vi "FY6900.vi"(4 "Error In":errorcluster, 7 "Command":T13) -> (0 "Error Out":errorcluster, 3 "Response":T11)   [LabVIEW 2018]
uses:
  MOKO_LabViewLibrary/MokoLowLevel/MokoLowLovelControl/MLLC_Command.ctl
  MOKO_LabViewLibrary/MokoLowLevel/MokoLowLovelControl/MLLC_Mode.ctl
  MOKO_LabViewLibrary/MokoLowLevel/MokoLowLovelControl/MLLC_Response.ctl
  MOKO_LabViewLibrary/MokoLowLevel/MokoLowLovelControl/MLLC_ConnectCluster.ctl
  MOKO_LabViewLibrary/MokoLowLevel/MokoLowLovelControl/MLLC_InterfaceType.ctl
  MOKO_LabViewLibrary/MokoLowLevel/MokoLowLovelControl/MLLC_OpenedSession.ctl
  MOKO_LabViewLibrary/MokoLowLevel/MokoLowLovelControl/MLLC_InterfaceSettings.ctl
  MOKO_LabViewLibrary/MokoLowLevel/MokoLowLovelControl/MLLC_InterfaceKind.ctl
  MOKO_LabViewLibrary/MokoLowLevel/MokoLowLovelControl/MLLC_DriverName.ctl
  MOKO_LabViewLibrary/MokoLowLevel/MokoLowLovelControl/MLLC_ResponseInit.ctl
  MOKO_LabViewLibrary/MokoLowLevel/MokoLowLovelControl/MLLC_Request.ctl
  MOKO_LabViewLibrary/MokoLowLevel/MokoLowLovelControl/MLLC_ErrorCode.ctl
  MOKO_LabViewLibrary/MokoLowLevel/MokoLowLovelControl/MLLC_Rs232Settings.ctl
panel:
  in  "Error Code":T1=5420
  in  "Request":T2="UMO"
  in  "ResponseInit":T3="FY6900"
  in  "Driver Name":T4="FY6900"
  in  "Settings":T10={"Saved Data"=variant, "Permanent data"={"Connect"={"InterfaceType"=enum."VISA", "OpenedSession"="", "InterfaceSettings"={"Interface"=enum."RS232", "EOS 4 read"=enum."LF (\\n)", "EOS 4 write"=enum."LF (\\n)", "TMO, ms"=2000, "Sett"=variant(cluster{"Baud Rate":u32, "Data Bits":u16, "Parity":u16, "Stop Bits":u16, "Flow Control":u16, "Eho":bool} {"Baud Rate"=75, "Data Bits"=0, "Parity"=0, "Stop Bits"=0, "Flow Control"=0, "Eho"=FALSE})}}}}
  in  "Mode":T12=enum."Check"
  # "FY6900"
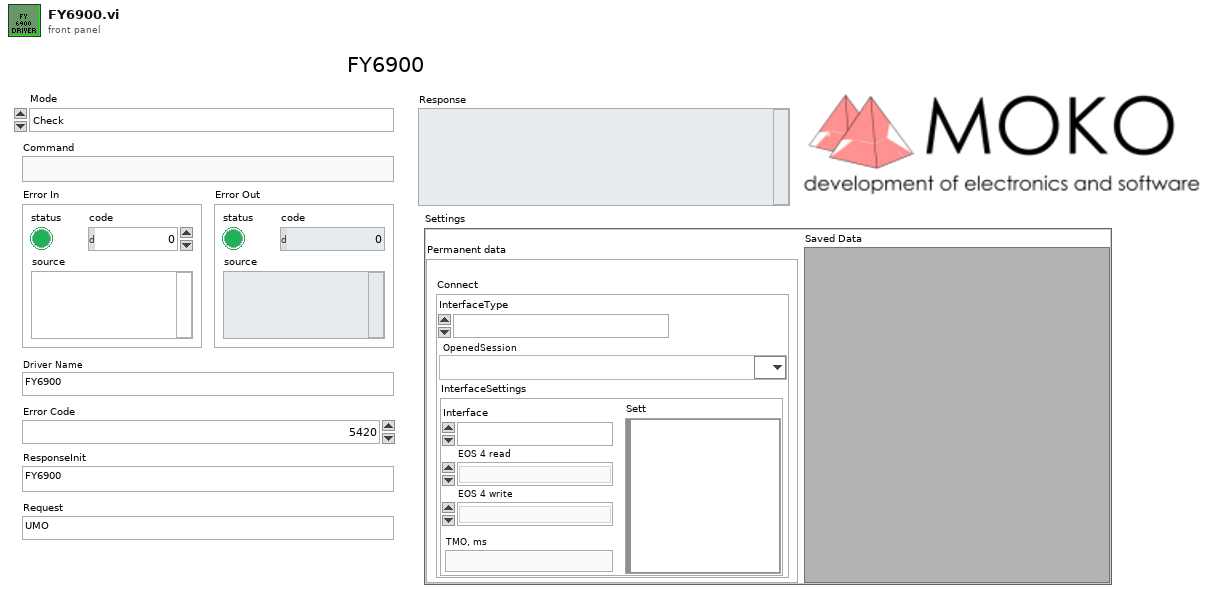
[diagram p1: front panel]
types:
  T1 = typedef "MLLC_ErrorCode.ctl" = u32
  T2 = typedef "MLLC_Request.ctl" = string
  T3 = typedef "MLLC_ResponseInit.ctl" = string
  T4 = typedef "MLLC_DriverName.ctl" = string
  T5 = typedef "MLLC_ConnectCluster.ctl" = cluster{"InterfaceType":T6, "OpenedSession":T7, "InterfaceSettings":T8}
  T6 = typedef "MLLC_InterfaceType.ctl" = enum16{"VISA", "Prologix USB-GPIB"}
  T7 = typedef "MLLC_OpenedSession.ctl" = refnum<visa-resource-name>
  T8 = typedef "MLLC_InterfaceSettings.ctl" = cluster{"Interface":T9, "EOS 4 read":enum16{"Default (=EOS 4 write)", "CR (\\r)", "LF (\\n)", "None"}, "EOS 4 write":enum16{"CR+LF (\\r\\n)", "CR (\\r)", "LF (\\n)", "None"}, "TMO, ms":i32, "Sett":variant}
  T9 = typedef "MLLC_InterfaceKind.ctl" = enum16{"RS232", "GPIB", "USB", "Ethernet", "another"}
  T10 = cluster{"Saved Data":variant, "Permanent data":cluster{"Connect":T5}}
  T11 = typedef "MLLC_Response.ctl" = string
  T12 = typedef "MLLC_Mode.ctl" = enum16{"get", "set", "close", "Init", "Check"}
  T13 = typedef "MLLC_Command.ctl" = string
  T14 = enum16{"CR+LF (\\r\\n)", "CR (\\r)", "LF (\\n)", "None"}
  T15 = enum16{"Default (=EOS 4 write)", "CR (\\r)", "LF (\\n)", "None"}
  T16 = typedef "MLLC_Error.ctl" = errorcluster
  T17 = typedef "MLLC_Rs232Settings.ctl" = cluster{"Baud Rate":u32, "Data Bits":u16, "Parity":u16, "Stop Bits":u16, "Flow Control":u16, "Eho":bool, "Address":dbl}
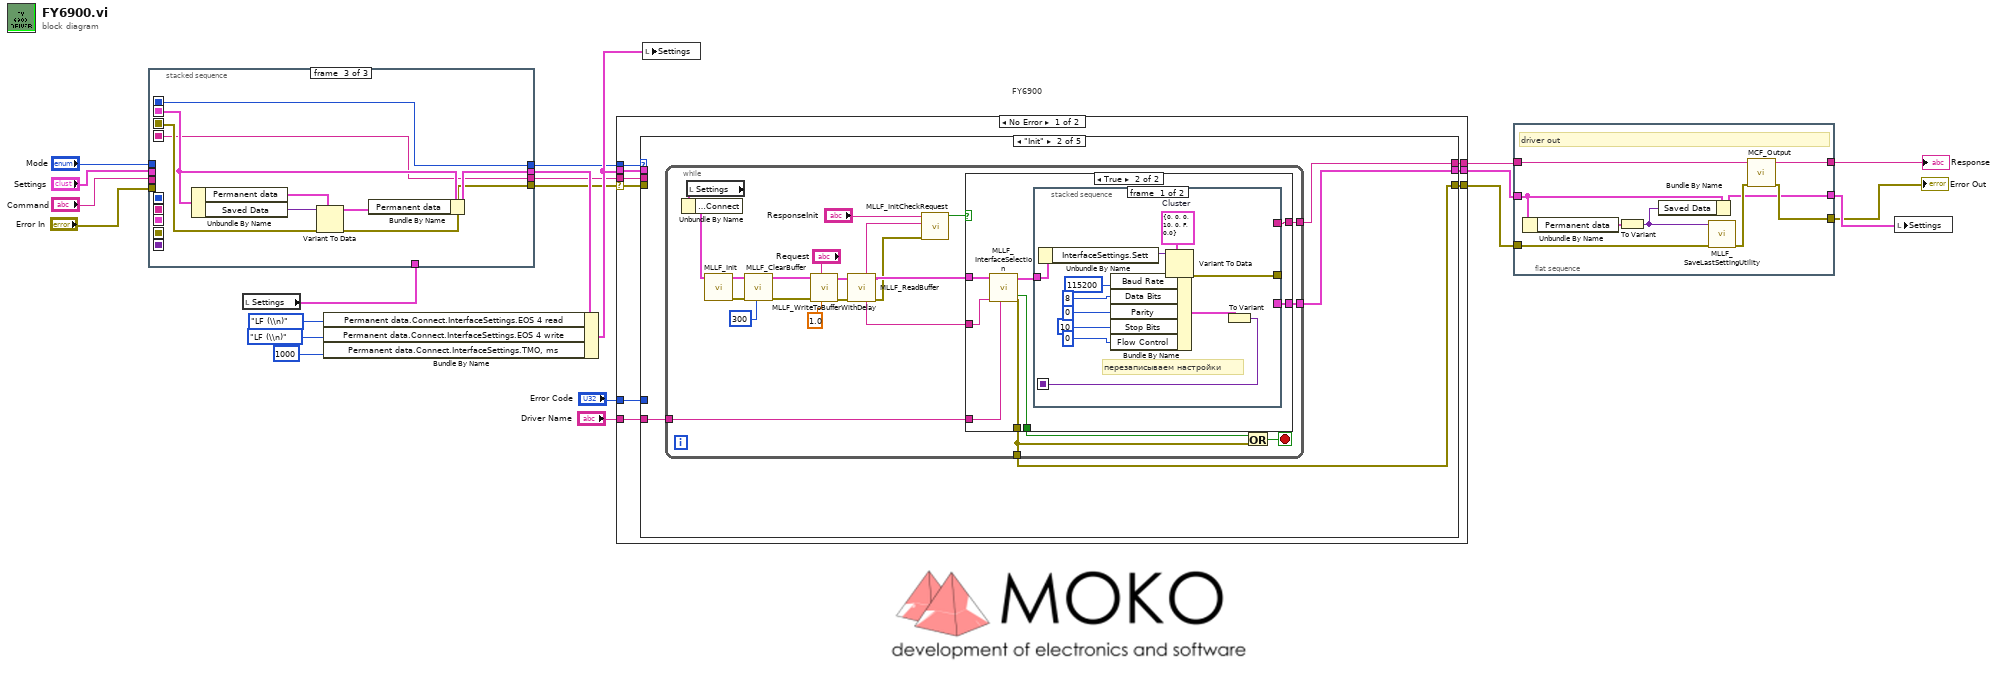
[diagram p0: block diagram]
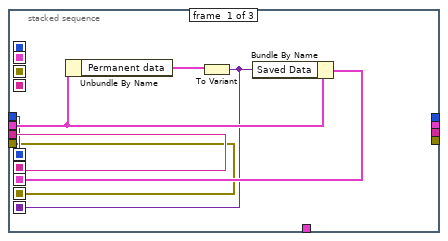
[diagram p2: hidden frame]
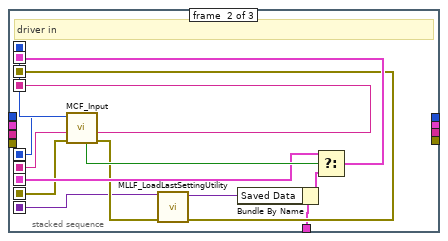
[diagram p3: hidden frame]
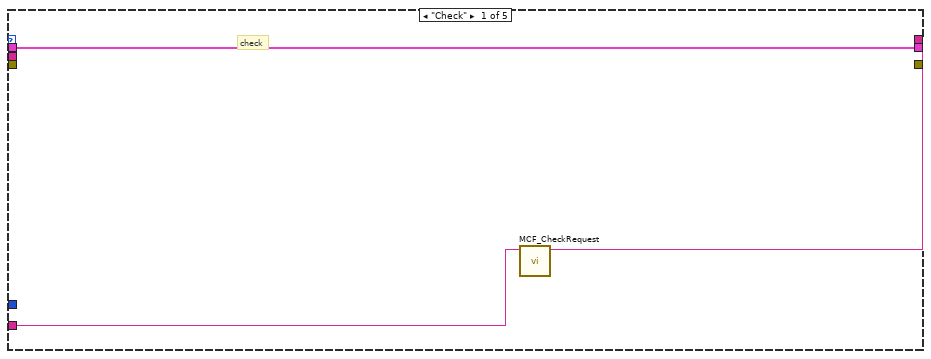
[diagram p4: hidden frame]
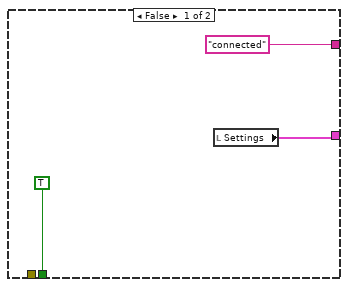
[diagram p5: hidden frame]
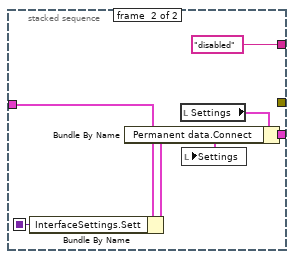
[diagram p6: hidden frame]
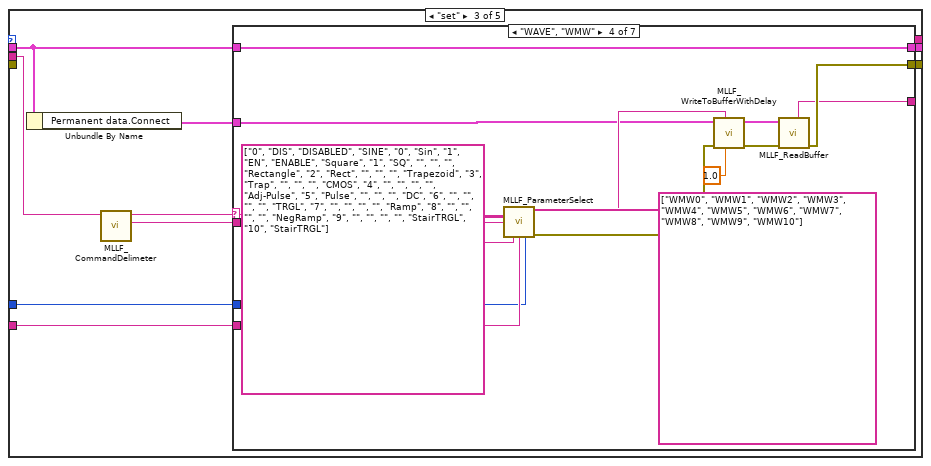
[diagram p7: hidden frame]
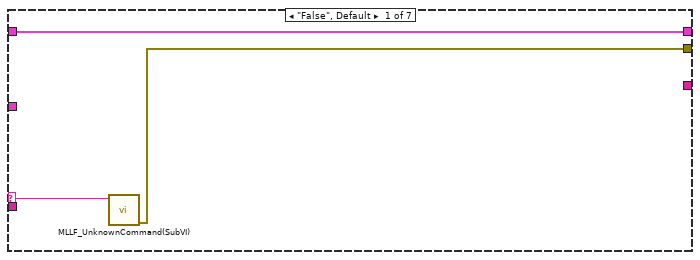
[diagram p8: hidden frame]
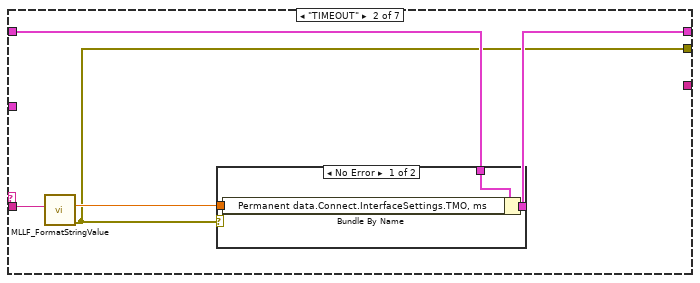
[diagram p9: hidden frame]
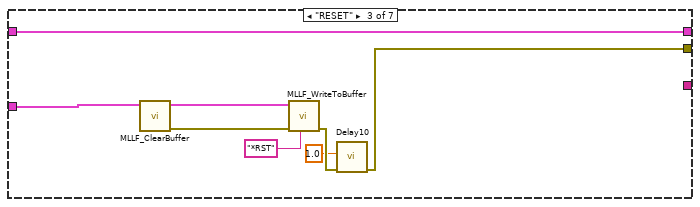
[diagram p11: hidden frame]
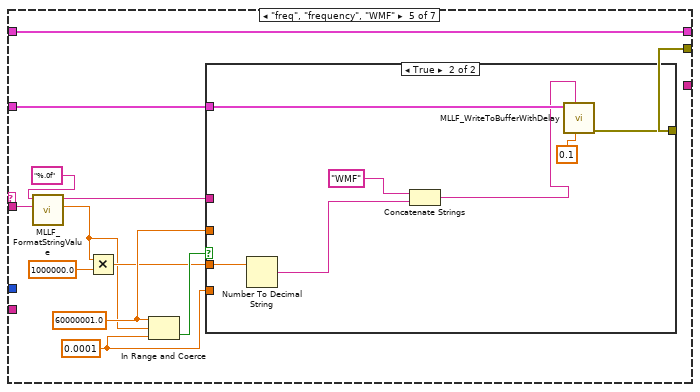
[diagram p12: hidden frame]
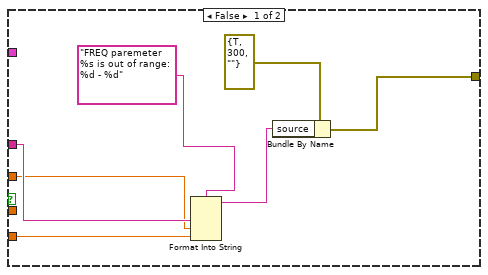
[diagram p13: hidden frame]
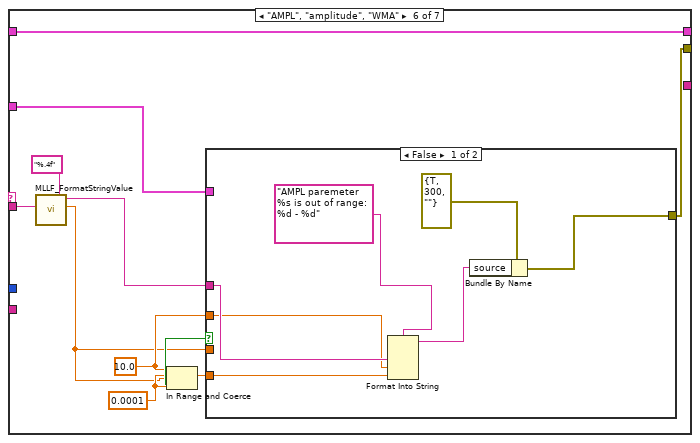
[diagram p14: hidden frame]
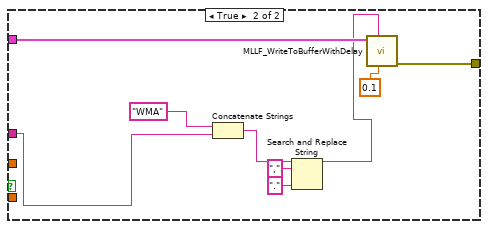
[diagram p15: hidden frame]
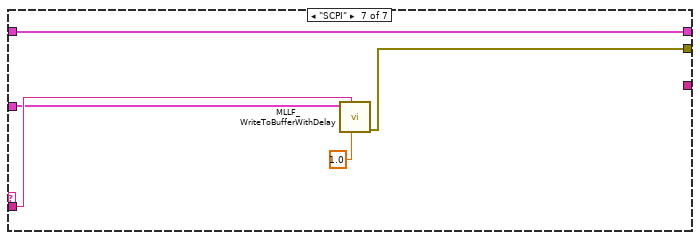
[diagram p16: hidden frame]
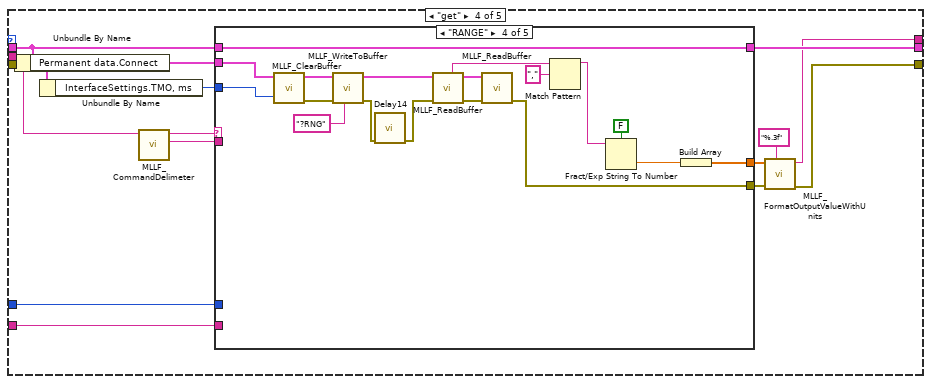
[diagram p17: hidden frame]
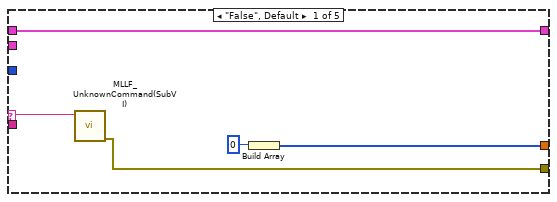
[diagram p18: hidden frame]
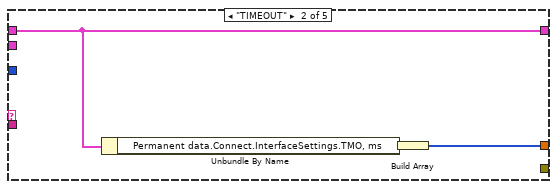
[diagram p19: hidden frame]
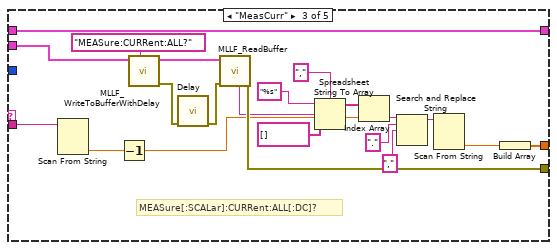
[diagram p20: hidden frame]
diagram:
  # "FY6900"
  n1 = local read "Settings"() -> (w5:T10)
  n2 = stacked-sequence {
    seq-local: [w24 _ _] -> [_ w40 _]
    seq-local: [w23 _ _] -> [_ w41 _]
    seq-local: [w26 _ _] -> [_ w36 _]
    seq-local: [w22 _ _] -> [_ w35 _]
    seq-local: [w25 _ _] -> [_ w31 _]
    seq-local: [_ w32 _] -> [_ _ w48]
    seq-local: [_ w42 _] -> [_ _ w45]
    seq-local: [_ w39 _] -> [_ _ w44]
    seq-local: [_ w38 _] -> [_ _ w49]
    tunnel: "Command" -> [w24 _ _]
    tunnel: "Mode" -> [w23 _ _]
    tunnel: "Error In" -> [w22 _ _]
    tunnel: "Settings" -> [w27 _ _]
    tunnel: w5 -> [_ w30 _]
    tunnel: [_ _ w44] -> w2
    tunnel: [_ _ w47] -> w4
    tunnel: [_ _ w46] -> w1
    tunnel: [_ _ w45] -> w3
    frame #0 {
      n3 = Unbundle By Name(w27) -> ("Permanent data"=w28:cluster{"Connect":T5})
      n4 = To Variant(anything=w28) -> (Variant=w25:variant)
      n5 = Bundle By Name(cluster=w27, "Saved Data"=w25) -> (w26:T10)
    }
    frame #1 {
      # "driver in"
      n6 = call "MCF_Input.vi"("Error In"=w35, "Command in"=w40, "Mode in"=w41) -> ("Error Out"=w34:errorcluster, "Command out"=w39:string, "Mode out"=w42:T12, "Boolean"=w37:bool)  [unwired: 5 in]
      n7 = call "MLLF_LoadLastSettingUtility.vi"("Error In"=w34, "Save data in"=w31) -> ("Error Out"=w32:errorcluster, "Save data out"=w29:variant)  [unwired: 8 in]
      n8 = Bundle By Name(cluster=w30, "Saved Data"=w29) -> (w33:T10)
      n9 = Select(t=w36, s=w37, f=w33) -> (s? t:f=w38:T10)
    }
    frame #2 {
      n10 = Unbundle By Name(w49) -> ("Permanent data"=w50:cluster{"Connect":T5}, "Saved Data"=w43:variant)
      n11 = Variant To Data(error in=w48, type=w50, Variant=w43) -> (data=w51:cluster{"Connect":T5}, error out=w46:errorcluster)
      n12 = Bundle By Name(cluster=w49, "Permanent data"=w51) -> (w47:T10)
    }
  }
  n13 = Bundle By Name(cluster=w4, "Permanent data.Connect.InterfaceSettings.EOS 4 read"=T15."LF (\\n)" ("Connect.InterfaceSettings.EOS 4 read"), "Permanent data.Connect.InterfaceSettings.EOS 4 write"=T14."LF (\\n)" ("Connect.InterfaceSettings.EOS 4 write"), "Permanent data.Connect.InterfaceSettings.TMO, ms"=1000 ("Connect.InterfaceSettings.TMO, ms")) -> (w19:T10)
  n14 = case shown="No Error" w1 {
    selector: w1 -> [w56 w304]
    tunnel: [w58 w304] -> w13
    tunnel: w3 -> [w60 _]
    tunnel: [w59 _] -> w15
    tunnel: w2 -> [w57 _]
    tunnel: w19 -> [w53 w303]
    tunnel: "Error Code" -> [w55 _]
    tunnel: "Driver Name" -> [w54 _]
    tunnel: [w52 w303] -> w14
    frame No Error {
      n15 = case shown="\"Init\"" w60 {
        tunnel: [w61 w65 _ w221 "" ("Output String")] -> w59
        tunnel: [_ w67 w122 w222 w301] -> w58
        tunnel: w57 -> [_ _ w121 w227 _]
        tunnel: w56 -> [_ _ _ _ _]
        tunnel: w55 -> [_ _ w127 w231 _]
        tunnel: w54 -> [w62 w64 w124 w230 _]
        tunnel: w53 -> [w63 _ w126 w233 w300]
        tunnel: [w63 w66 w125 w232 w300] -> w52
        frame "Check" {
          # "check"
          n16 = call "MCF_CheckRequest.vi"("Driver Name"=w62) -> ("Output String"=w61:string)  [unwired: 9 in, 1 out]
        }
        frame "Init" {
          n17 = while {
            tunnel: [w83] -> w67
            tunnel: [w80] -> w66
            tunnel: [w79] -> w65
            tunnel: w64 -> [w73]
            stop <- w85 stop-if-true
            n18 = local read "Settings"() -> (w89:T10)
            n19 = Unbundle By Name(w89) -> ("Permanent data.Connect"=w86:T5)
            n20 = call "MLLF_Init.vi"("DriverConnect in"=w86) -> ("Error Out"=w75:errorcluster, "DriverConnect out"=w76:T5)  [unwired: 7 in]
            n21 = call "MLLF_ClearBuffer.vi"("Timeout(default = 300 ms)"=u32 300 ("Timeout"), "Error In"=w75, "DriverConnect in"=w76) -> ("Error Out"=w71:errorcluster, "DriverConnect out"=w72:T5)  [unwired: 5 in, 1 out]
            n22 = call "MLLF_WriteToBufferWithDelay.vi"("Delay Time ( 0,05 s)"=1.0 ("Delay Time (s)"), "Command"="Request", "Error In"=w71, "DriverConnect in"=w72) -> ("Error Out"=w82:errorcluster, "DriverConnect out"=w88:T5)  [unwired: 6 in]
            n23 = call "MLLF_ReadBuffer.vi"("Error In"=w82, "DriverConnect in"=w88) -> ("Error Out"=w69:errorcluster, "DriverConnect out"=w70:T5, "String"=w68:string)  [unwired: 6 in]
            n24 = call "MLLF_InitCheckRequest.vi"("error in (no error)"=w69, "Answer"=w68, "Response Init"="ResponseInit") -> ("Design"=w77:bool)  [unwired: 5 in, 3 out]
            n25 = case shown="True" w77 {
              tunnel: w70 -> [_ w99]
              tunnel: [TRUE w95] -> w84
              tunnel: [_ w100] -> w83
              tunnel: [w90 w97] -> w80
              tunnel: ["connected" w96] -> w79
              tunnel: w68 -> [_ w93]
              tunnel: w73 -> [_ w94]
              frame False {
                n26 = local read "Settings"() -> (w90:T10)
              }
              frame True {
                n27 = call "MLLF_InterfaceSelection.vi"("Driver Name"=w94, "Answer:"=w93, "DriverConnect in"=w99) -> ("error out"=w100:T16, "DriverConnect out"=w98:T5, "stop init?"=w95:bool)  [unwired: 4 in, 2 out]
                n28 = stacked-sequence {
                  seq-local: [w103 _] -> [_ w117]
                  tunnel: w98 -> [w102 w114]
                  tunnel: [w104 _] -> _
                  tunnel: [_ w116] -> w97
                  tunnel: [_ "disabled"] -> w96
                  frame #0 {
                    w106 = T17 {"Baud Rate"=0, "Data Bits"=0, "Parity"=0, "Stop Bits"=10, "Flow Control"=0, "Eho"=FALSE, "Address"=0.0}  # Cluster
                    # "перезаписываем настройки"
                    n29 = Unbundle By Name(w102) -> ("InterfaceSettings.Sett"=w105:variant)
                    n30 = Variant To Data(type=w106, Variant=w105) -> (data=w107:T17, error out=w104:errorcluster)  [unwired: 1 in]
                    n31 = Bundle By Name(cluster=w107, "Baud Rate"=u32 115200, "Data Bits"=u16 8 ("Serial Settings:Data Bits"), "Parity"=u16 0 ("Serial Settings:Parity"), "Stop Bits"=u16 10 ("Serial Settings:Stop Bits"), "Flow Control"=u16 0 ("Serial Settings:Flow Control")) -> (w112:T17)
                    n32 = To Variant(anything=w112) -> (Variant=w103:variant)
                  }
                  frame #1 {
                    n33 = Bundle By Name(cluster=w114, "InterfaceSettings.Sett"=w117) -> (w113:T5)
                    n34 = local read "Settings"() -> (w118:T10)
                    n35 = Bundle By Name(cluster=w118, "Permanent data.Connect"=w113) -> (w116:T10)
                    n36 = local write "Settings"(w116) -> ()
                  }
                }
              }
            }
            n37 = Or(x=w84, y=w83) -> (x .or. y?=w85:bool)
          }
        }
        frame "set" {
          n38 = Unbundle By Name(w126) -> ("Permanent data.Connect"=w123:T5)
          n39 = call "MLLF_CommandDelimeter.vi"("command with param"=w121) -> ("param 1"=w119:string, "command"=w120:string)  [unwired: 6 in, 3 out]
          n40 = case shown="\"WAVE\", \"WMW\"" w120 {
            selector: w120 -> [w129 _ _ w152 _ _ _]
            tunnel: w119 -> [_ w133 _ w161 w170 w194 w217]
            tunnel: w127 -> [_ _ _ w157 _ _ _]
            tunnel: w126 -> [w130 w134 w147 w162 w163 w189 w219]
            tunnel: [w130 w135 w147 w162 w163 w189 w219] -> w125
            tunnel: w123 -> [_ _ w145 w153 w169 w190 w216]
            tunnel: w124 -> [_ _ _ w158 _ _ _]
            tunnel: [w128 w131 w140 w149 w168 w193 w215] -> w122
            tunnel: [_ _ _ w148 _ _ _] -> _
            frame "False", Default {
              n41 = call "MLLF_UnknownCommand(SubVI).vi"("Unknown command"=w129) -> ("error out"=w128:errorcluster)  [unwired: 10 in]
            }
            frame "TIMEOUT" {
              n42 = call "MLLF_FormatStringValue.vi"("String Value"=w133) -> ("error out"=w131:T16, "number"=w132:dbl)  [unwired: 8 in, 1 out]
              n43 = case shown="No Error" w131 {
                tunnel: [w138 w139] -> w135
                tunnel: w134 -> [w137 w139]
                tunnel: w132 -> [w136 _]
                frame No Error {
                  n44 = Bundle By Name(cluster=w137, "Permanent data.Connect.InterfaceSettings.TMO, ms"=w136) -> (w138:T10)
                }
                frame Error {
                }
              }
            }
            frame "RESET" {
              n45 = call "MLLF_ClearBuffer.vi"("DriverConnect in"=w145) -> ("Error Out"=w144:errorcluster, "DriverConnect out"=w143:T5)  [unwired: 7 in, 1 out]
              n46 = call "MLLF_WriteToBuffer.vi"("String"="*RST", "error in"=w144, "DriverConnect in"=w143) -> ("error out"=w142:T16)  [unwired: 5 in, 1 out]
              n47 = call "Delay10"("error in (no error)"=w142, "Delay Time (s)"=1.0) -> ("error out"=w140:errorcluster)  [unwired: 9 in]
            }
            frame "WAVE", "WMW" {
              n48 = call "MLLF_ParameterSelect.vi"("Command to equipment"=string[] ["WMW0", "WMW1", "WMW2", "WMW3", "WMW4", "WMW5", "WMW6", "WMW7", "WMW8", "WMW9", "WMW10"] ("Names"), "Names"=string[][] [["0", "DIS", "DISABLED", "SINE", "0", "Sin"], ["1", "EN", "ENABLE", "Square", "1", "SQ"], ["", "", "", "Rectangle", "2", "Rect"], ["", "", "", "Trapezoid", "3", "Trap"], ["", "", "", "CMOS", "4", ""], ["", "", "", "Adj-Pulse", "5", "Pulse"], ["", "", "", "DC", "6", ""], ["", "", "", "TRGL", "7", ""], ["", "", "", "Ramp", "8", ""], ["", "", "", "NegRamp", "9", ""], ["", "", "", "StairTRGL", "10", "StairTRGL"]], "Input"=w161, "Command"=w152, "Driver Name"=w158, "Error Code"=w157) -> ("Choice"=w154:string, "Error Out"=w155:errorcluster)  [unwired: 8 in]
              n49 = call "MLLF_WriteToBufferWithDelay.vi"("Delay Time ( 0,05 s)"=1.0 ("Delay Time (s)"), "Command"=w154, "Error In"=w155, "DriverConnect in"=w153) -> ("Error Out"=w151:errorcluster, "DriverConnect out"=w150:T5)  [unwired: 6 in]
              n50 = call "MLLF_ReadBuffer.vi"("Error In"=w151, "DriverConnect in"=w150) -> ("Error Out"=w149:errorcluster, "String"=w148:string)  [unwired: 6 in, 1 out]
            }
            frame "freq", "frequency", "WMF" {
              w172 = 0.0001 ("lower limit")
              w171 = 60000001.0 ("upper limit")
              n51 = call "MLLF_FormatStringValue.vi"("String Value"=w170, "Format"=T13 "%.0f") -> ("number"=w164:dbl, "String Value Formated"=w173:T13)  [unwired: 7 in, 1 out]
              n52 = Multiply(x=w164, y=1000000.0) -> (x*y=w165:dbl)
              n53 = In Range and Coerce(upper limit=w171, x=w164, lower limit=w172) -> (In Range?=w174:bool)  [unwired: 1 out]
              n54 = case shown="True" w174 {
                tunnel: w169 -> [_ w187]
                tunnel: [w180 w184] -> w168
                tunnel: w173 -> [w179 _]
                tunnel: w172 -> [w176 _]
                tunnel: w171 -> [w175 _]
                tunnel: w165 -> [_ w183]
                frame False {
                  n55 = Format Into String(format string="FREQ paremeter %s is out of range: %d - %d", w179, w175, w176) -> (resulting string=w178:string)  [unwired: 2 in, 1 out]
                  n56 = Bundle By Name(cluster=errorcluster {"status"=TRUE, "code"=300, "source"=""} ("Error Out"), "source"=w178) -> (w180:errorcluster)
                }
                frame True {
                  n57 = Number To Decimal String(number=w183) -> (decimal integer string=w182:string)  [unwired: 1 in]
                  n58 = Concatenate Strings(T13 "WMF" ("Command"), w182) -> (w186:string)
                  n59 = call "MLLF_WriteToBufferWithDelay.vi"("Delay Time ( 0,05 s)"=0.1 ("Delay Time (s)"), "Command"=w186, "DriverConnect in"=w187) -> ("Error Out"=w184:errorcluster)  [unwired: 7 in, 1 out]
                }
              }
            }
            frame "AMPL", "amplitude", "WMA" {
              w196 = 0.0001 ("lower limit")
              w195 = 10.0 ("upper limit")
              n60 = call "MLLF_FormatStringValue.vi"("String Value"=w194, "Format"=T13 "%.4f") -> ("number"=w191:dbl, "String Value Formated"=w197:T13)  [unwired: 7 in, 1 out]
              n61 = In Range and Coerce(upper limit=w195, x=w191, lower limit=w196) -> (In Range?=w198:bool)  [unwired: 1 out]
              n62 = case shown="False" w198 {
                tunnel: w190 -> [_ w213]
                tunnel: [w204 w211] -> w193
                tunnel: w197 -> [w203 w210]
                tunnel: w196 -> [w200 _]
                tunnel: w195 -> [w199 _]
                tunnel: w191 -> [_ _]
                frame False {
                  n63 = Format Into String(format string="AMPL paremeter %s is out of range: %d - %d", w203, w199, w200) -> (resulting string=w202:string)  [unwired: 2 in, 1 out]
                  n64 = Bundle By Name(cluster=errorcluster {"status"=TRUE, "code"=300, "source"=""} ("Error Out"), "source"=w202) -> (w204:errorcluster)
                }
                frame True {
                  n65 = Concatenate Strings(T13 "WMA" ("Command"), w210) -> (w209:string)
                  n66 = Search and Replace String(input string=w209, search string=",", replace string="." ("replace string (\"\")")) -> (result string=w206:string)  [unwired: 5 in, 3 out]
                  n67 = call "MLLF_WriteToBufferWithDelay.vi"("Delay Time ( 0,05 s)"=0.1 ("Delay Time (s)"), "Command"=w206, "DriverConnect in"=w213) -> ("Error Out"=w211:errorcluster)  [unwired: 7 in, 1 out]
                }
              }
            }
            frame "SCPI" {
              n68 = call "MLLF_WriteToBufferWithDelay.vi"("Delay Time ( 0,05 s)"=1.0 ("Delay Time (s)"), "Command"=w217, "DriverConnect in"=w216) -> ("Error Out"=w215:errorcluster)  [unwired: 7 in, 1 out]
            }
          }
        }
        frame "get" {
          n69 = Unbundle By Name(w233) -> ("Permanent data.Connect"=w224:T5)
          n70 = Unbundle By Name(w224) -> ("InterfaceSettings.TMO, ms"=w223:i32)
          n71 = call "MLLF_CommandDelimeter.vi"("command with param"=w227) -> ("param 1"=w225:string, "command"=w226:string)  [unwired: 6 in, 3 out]
          n72 = case shown="\"RANGE\"" w226 {
            selector: w226 -> [w235 _ _ _ _]
            tunnel: w225 -> [_ _ w252 _ _]
            tunnel: [w234 _ w257 w271 w289] -> w229
            tunnel: w231 -> [_ _ _ _ _]
            tunnel: [w238 w241 w262 w280 w298] -> w232
            tunnel: w233 -> [w238 w241 w262 w280 w298]
            tunnel: [w236 w239 w261 w277 w295] -> w228
            tunnel: w224 -> [_ _ w242 w275 w293]
            tunnel: w230 -> [_ _ _ _ _]
            tunnel: w223 -> [_ _ _ w274 w292]
            frame "False", Default {
              n73 = call "MLLF_UnknownCommand(SubVI).vi"("Unknown command"=w235) -> ("error out"=w234:errorcluster)  [unwired: 10 in]
              n74 = Build Array(0 ("TimeOut")) -> (w236:i32[])
            }
            frame "TIMEOUT" {
              n75 = Unbundle By Name(w241) -> ("Permanent data.Connect.InterfaceSettings.TMO, ms"=w240:i32)
              n76 = Build Array(w240) -> (w239:i32[])
            }
            frame "MeasCurr" {
              # "MEASure[:SCALar]:CURRent:ALL[:DC]?"
              n77 = Scan From String(input string=w252) -> (output 1=w247:dbl)  [unwired: 4 in, 3 out]
              n78 = Decrement(x=w247) -> (x-1=w246:dbl)
              n79 = call "MLLF_WriteToBufferWithDelay.vi"("Command"="MEASure:CURRent:ALL?" ("String"), "DriverConnect in"=w242) -> ("Error Out"=w259:errorcluster, "DriverConnect out"=w243:T5)  [unwired: 8 in]
              n80 = call "Delay"("error in (no error)"=w259) -> ("error out"=w258:errorcluster)  [unwired: 10 in]
              n81 = call "MLLF_ReadBuffer.vi"("Error In"=w258, "DriverConnect in"=w243) -> ("Error Out"=w257:errorcluster, "String"=w251:string)  [unwired: 6 in, 1 out]
              n82 = Spreadsheet String To Array(delimiter (Tab)=",", format string="%s", spreadsheet string=w251, array type (2D Dbl)=string[] [] ("appended array")) -> (array=w256:string[])
              n83 = Index Array(array=w256, index=w246) -> (element=w250:string)
              n84 = Search and Replace String(input string=w250, search string=".", replace string="," ("replace string (\"\")")) -> (result string=w245:string)  [unwired: 5 in, 3 out]
              n85 = Scan From String(input string=w245) -> (output 1=w244:dbl)  [unwired: 4 in, 3 out]
              n86 = Build Array(w244) -> (w261:dbl[])
            }
            frame "RANGE" {
              n87 = call "MLLF_ClearBuffer.vi"("Timeout(default = 300 ms)"=w274, "DriverConnect in"=w275) -> ("Error Out"=w272:errorcluster, "DriverConnect out"=w273:T5)  [unwired: 6 in, 1 out]
              n88 = call "MLLF_WriteToBuffer.vi"("String"="?RNG", "error in"=w272, "DriverConnect in"=w273) -> ("error out"=w264:T16, "DriverConnect out"=w268:T5)  [unwired: 5 in]
              n89 = call "Delay14"("error in (no error)"=w264) -> ("error out"=w263:errorcluster)  [unwired: 10 in]
              n90 = call "MLLF_ReadBuffer.vi"("Error In"=w263, "DriverConnect in"=w268) -> ("Error Out"=w267:errorcluster, "DriverConnect out"=w266:T5, "String"=w265:string)  [unwired: 6 in]
              n91 = call "MLLF_ReadBuffer.vi"("Error In"=w267, "DriverConnect in"=w266) -> ("Error Out"=w271:errorcluster)  [unwired: 6 in, 2 out]
              n92 = Match Pattern(string=w265, regular expression=",") -> (before substring=w269:string)  [unwired: 1 in, 3 out]
              n93 = Fract/Exp String To Number(use system decimal point (T)=FALSE, string=w269) -> (number=w278:dbl)  [unwired: 2 in, 1 out]
              n94 = Build Array(w278) -> (w277:dbl[])
            }
            frame "ZERO" {
              n95 = call "MLLF_ClearBuffer.vi"("Timeout(default = 300 ms)"=w292, "DriverConnect in"=w293) -> ("Error Out"=w290:errorcluster, "DriverConnect out"=w291:T5)  [unwired: 6 in, 1 out]
              n96 = call "MLLF_WriteToBuffer.vi"("String"="?Z,U", "error in"=w290, "DriverConnect in"=w291) -> ("error out"=w282:T16, "DriverConnect out"=w286:T5)  [unwired: 5 in]
              n97 = call "Delay15"("error in (no error)"=w282) -> ("error out"=w281:errorcluster)  [unwired: 10 in]
              n98 = call "MLLF_ReadBuffer.vi"("Error In"=w281, "DriverConnect in"=w286) -> ("Error Out"=w285:errorcluster, "DriverConnect out"=w284:T5, "String"=w283:string)  [unwired: 6 in]
              n99 = call "MLLF_ReadBuffer.vi"("Error In"=w285, "DriverConnect in"=w284) -> ("Error Out"=w289:errorcluster)  [unwired: 6 in, 2 out]
              n100 = Match Pattern(string=w283, regular expression=",") -> (before substring=w287:string)  [unwired: 1 in, 3 out]
              n101 = Fract/Exp String To Number(use system decimal point (T)=FALSE, string=w287) -> (number=w296:dbl)  [unwired: 2 in, 1 out]
              n102 = Build Array(w296) -> (w295:dbl[])
            }
          }
          n103 = call "MLLF_FormatOutputValueWithUnits.vi"("Format"=T13 "%.3f", "error in"=w229, "ValuesIn"=w228) -> ("error out"=w222:T16, "Result string"=w221:T13)  [unwired: 7 in]
        }
        frame "close" {
          n104 = Unbundle By Name(w300) -> ("Permanent data.Connect.OpenedSession"=w302:T7)
          n105 = VISA Close(VISA resource name=w302) -> (error out=w301:errorcluster)  [unwired: 1 in]
        }
      }
    }
    frame Error {
    }
  }
  n106 = local write "Settings"(w19) -> ()
  n107 = flat-sequence {
    tunnel: [w313] -> w12
    tunnel: [w312] -> w10
    tunnel: w15 -> [w311]
    tunnel: w13 -> [w310]
    tunnel: w14 -> [w306]
    tunnel: [w308] -> w11
    frame #0 {
      # "driver out"
      n108 = Unbundle By Name(w306) -> ("Permanent data"=w305:cluster{"Connect":T5})
      n109 = To Variant(anything=w305) -> (Variant=w307:variant)
      n110 = Bundle By Name(cluster=w306, "Saved Data"=w307) -> (w308:T10)
      n111 = call "MLLF_SaveLastSettingUtility.vi"("error in"=w310, "Saved Data"=w307) -> ("error out"=w309:T16)  [unwired: 8 in, 1 out]
      n112 = call "MCF_Output.vi"("Error In"=w309, "Input"=w311) -> ("Error Out"=w312:errorcluster, "Output"=w313:string)  [unwired: 8 in]
    }
  }
  n113 = local write "Settings"(w11) -> ()
  "Response" <- w12
  "Error Out" <- w10
